vi "Parse Sentence.vi"(8 "error in (no error)":errorcluster, 11 "Ocean Server Sentence":string) -> (0 "error out":errorcluster, 3 "Values":T1)   [LabVIEW 2011, in "Ocean Server OS4000.lvlib"]
doc: "Parses the sentence and outputs the data."
uses:
  Ocean Server OS4000.lvlib
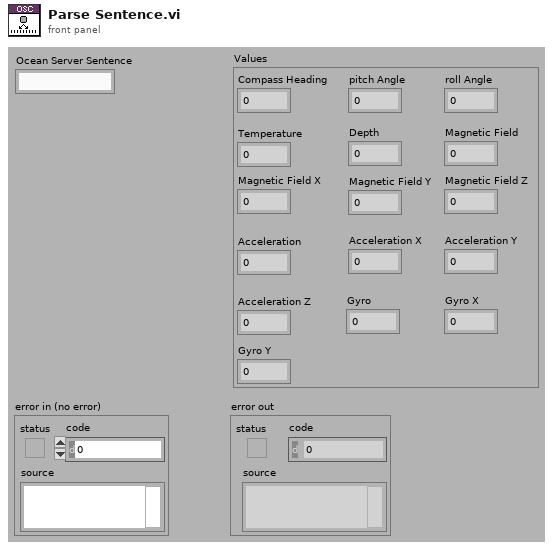
[diagram p1: front panel]
types:
  T1 = cluster{"Compass Heading":dbl, "pitch Angle":dbl, "roll Angle":dbl, "Temperature":dbl, "Depth":dbl, "Magnetic Field":dbl, "Magnetic Field X":dbl, "Magnetic Field Y":dbl, "Magnetic Field Z":dbl, "Acceleration":dbl, "Acceleration X":dbl, "Acceleration Y":dbl, "Gyro":dbl, "Gyro X":dbl, "Acceleration Z":dbl, "Gyro Y":dbl}
  T2 = cluster{"Compass Heading":dbl, "pitchAngle":dbl, "rollAngle":dbl, "Temperature":dbl, "Depth":dbl, "Magnetic Field":dbl, "Magnetic Field X":dbl, "Magnetic Field Y":dbl, "Magnetic Field Z":dbl, "Acceleration":dbl, "Acceleration X":dbl, "Acceleration Y":dbl, "Gyro":dbl, "Gyro X":dbl, "Acceleration Z":dbl, "Gyro Y":dbl}
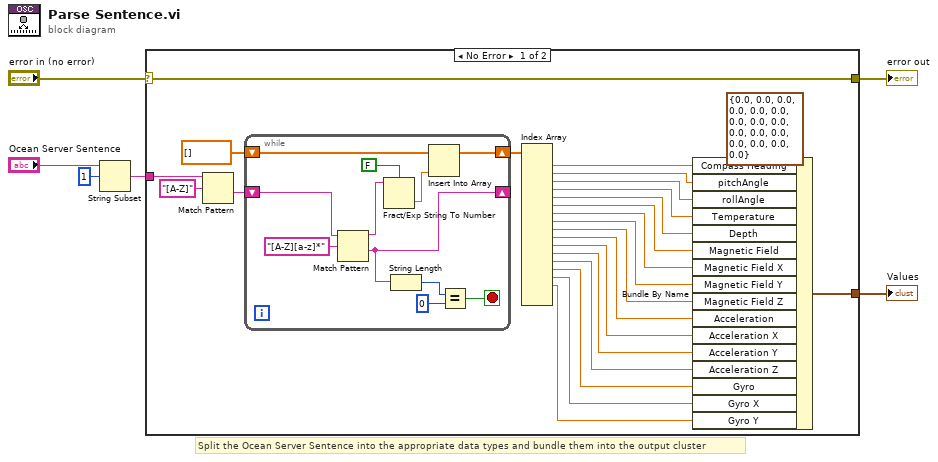
[diagram p0: block diagram]
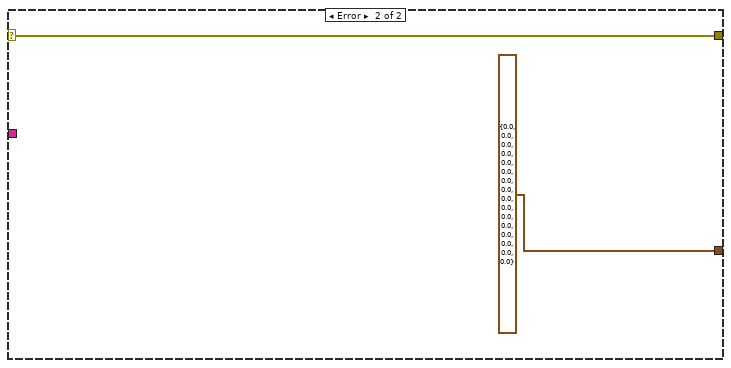
[diagram p2: hidden frame]
diagram:
  # "Split the Ocean Server Sentence into the appropriate data types and bundle them into the output cluster"
  n1 = String Subset(string="Ocean Server Sentence", offset (0)=1) -> (substring=w4:string)  [unwired: 1 in]
  n2 = case shown="No Error" "error in (no error)" {
    selector: "error in (no error)" -> [w8 w43]
    tunnel: w4 -> [w28 _]
    tunnel: [w8 w43] -> w5
    tunnel: [w7 T2 {"Compass Heading"=0.0, "pitchAngle"=0.0, "rollAngle"=0.0, "Temperature"=0.0, "Depth"=0.0, "Magnetic Field"=0.0, "Magnetic Field X"=0.0, "Magnetic Field Y"=0.0, "Magnetic Field Z"=0.0, "Acceleration"=0.0, "Acceleration X"=0.0, "Acceleration Y"=0.0, "Gyro"=0.0, "Gyro X"=0.0, "Acceleration Z"=0.0, "Gyro Y"=0.0} ("Data")] -> w1
    frame No Error {
      n3 = Match Pattern(string=w28, regular expression="[A-Z]") -> (after substring=w27:string)  [unwired: 1 in, 3 out]
      n4 = while {
        shift-right: [w37] -> w26
        shift-left: dbl[] [] ("array") -> [w38]
        shift-right: [w36] -> _
        shift-left: w27 -> [w32]
        stop <- w33 stop-if-true
        n5 = Match Pattern(string=w32, regular expression="[A-Z][a-z]*") -> (before substring=w40:string, after substring=w36:string)  [unwired: 1 in, 2 out]
        n6 = Fract/Exp String To Number(use system decimal point (T)=FALSE, string=w40) -> (number=w39:dbl)  [unwired: 2 in, 1 out]
        n7 = String Length(string=w36) -> (length=w35:i32)
        n8 = Insert Into Array(array=w38, new element=w39) -> (w37:dbl[])  [unwired: 1 in]
        n9 = Equal?(x=w35, y=0) -> (x = y?=w33:bool)
      }
      n10 = Index Array(array=w26) -> (element #1=w24:dbl, element #2=w23:dbl, element #3=w22:dbl, element #4=w21:dbl, element #5=w20:dbl, element #6=w19:dbl, element #7=w18:dbl, element #8=w17:dbl, element #9=w16:dbl, element #10=w15:dbl, element #11=w14:dbl, element #12=w13:dbl, element #13=w12:dbl, element #14=w11:dbl, element #15=w10:dbl, element #16=w9:dbl)  [unwired: 18 in, 2 out]
      n11 = Bundle By Name(cluster=T2 {"Compass Heading"=0.0, "pitchAngle"=0.0, "rollAngle"=0.0, "Temperature"=0.0, "Depth"=0.0, "Magnetic Field"=0.0, "Magnetic Field X"=0.0, "Magnetic Field Y"=0.0, "Magnetic Field Z"=0.0, "Acceleration"=0.0, "Acceleration X"=0.0, "Acceleration Y"=0.0, "Gyro"=0.0, "Gyro X"=0.0, "Acceleration Z"=0.0, "Gyro Y"=0.0} ("Data"), "Compass Heading"=w24, "pitchAngle"=w23, "rollAngle"=w22, "Temperature"=w21, "Depth"=w20, "Magnetic Field"=w19, "Magnetic Field X"=w18, "Magnetic Field Y"=w17, "Magnetic Field Z"=w16, "Acceleration"=w15, "Acceleration X"=w14, "Acceleration Y"=w13, "Acceleration Z"=w12, "Gyro"=w11, "Gyro X"=w10, "Gyro Y"=w9) -> (w7:T2)
    }
    frame Error {
    }
  }
  "error out" <- w5
  "Values" <- w1
